vi "FT_Set_Flow_Control.vi"(2 "XOff":u8 format="%x", 3 "XOn":u8 format="%x", 4 "Flow Control":u16(ring) items=["None"=0, "RTS-CTS"=256, "DTR-DSR"=512, "XOn-XOff"=1024], 5 "Handle":u32) -> (0 "FT_Status":u32, 1 "Handle 2":u32)   [LabVIEW 2011]
uses:
  FTD2XX.dll
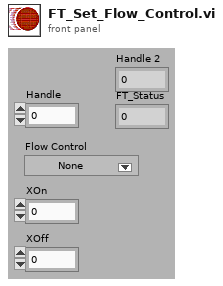
[diagram p1: front panel]
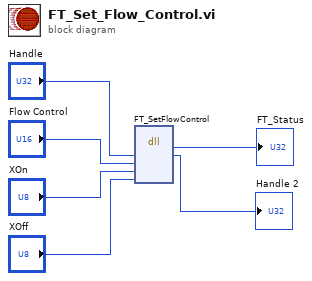
[diagram p0: block diagram]
diagram:
  n1 = dll-call lib="D:/WORK/LabView/#Avesta/D2XX_Functions_7.0/FTD2XX.dll" fn="FT_SetFlowControl"("Handle"="Handle", "FlowControl"="Flow Control", "XOn"="XOn", "XOff"="XOff") -> ("FT_Status"=→"FT_Status":u32, "Handle"=→"Handle 2":u32)  [unwired: 6 in, 2 out]
